vi "Enable Multiple Boolean Controls.vi"(8 "error in":errorcluster, 10 "Enabled":bool=TRUE, 11 "References":refnum<vi>[](array[refnum])) -> (0 "error out":errorcluster)   [LabVIEW 2015]
doc: "Enables or disables group of UI controls"
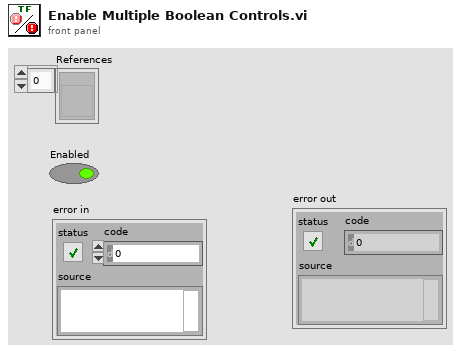
[diagram p1: front panel]
types:
  T1 = enum8{"Enabled", "Disabled", "Disabled and Grayed Out"}
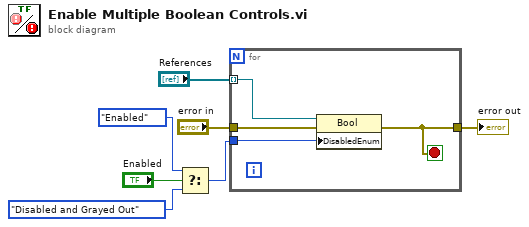
[diagram p0: block diagram]
diagram:
  n1 = Select(t=T1."Enabled" ("Disabled"), s="Enabled", f=T1."Disabled and Grayed Out" ("Disabled")) -> (s? t:f=w3:T1)
  n2 = for {
    tunnel: "References" -> [w11] mode=indexing
    tunnel: w3 -> [w10]
    tunnel: "error in" -> [w9]
    tunnel: [w8] -> w1
    stop <- w8 stop-if-true
    n3 = property class="Bool"(reference=w11, error in=w9, "DisabledEnum"=w10) -> (error out=w8:errorcluster)  [unwired: 1 out]
  }
  "error out" <- w1
